vi "rs3 create frame queue.vi"(8 "error in (no error)":errorcluster, 11 "capacity":i32=2) -> (0 "error out":errorcluster, 1 "error":u64, 2 "queue":u64)   [LabVIEW 2017, in "libRealSense3.lvlib"]
doc: "Creates a Frame Queue that will be used to CAPTURE streams with. \nThis QUEUE goes into the START QUEUE and Wait_for_Frames VI.\n\nThe capacity should generally be at least as large as the number of streams configured to stream."
uses:
  libRealSense3.lvlib
  realsense2.dll
panel:
  # "RS3 Create Frame Queue"
  # "(C) Intel Corp.,  AGJ"
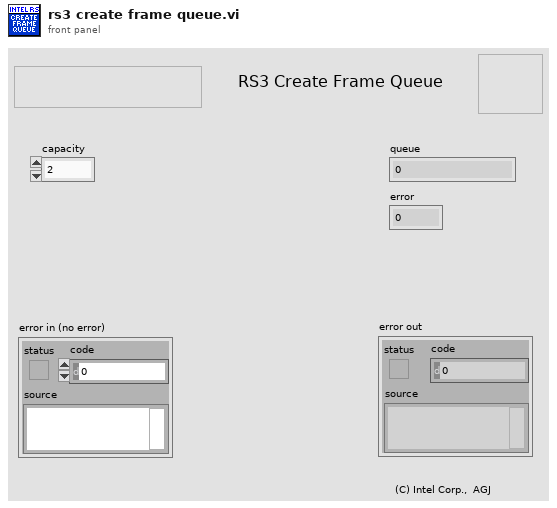
[diagram p1: front panel]
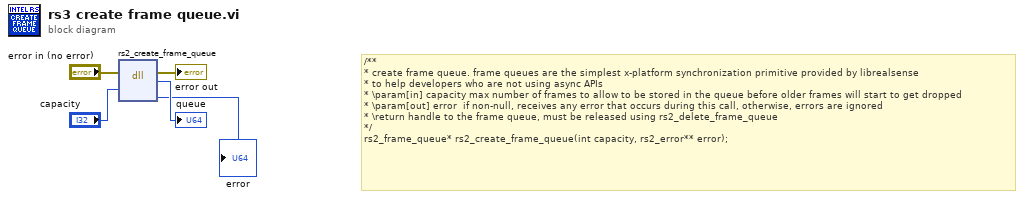
[diagram p0: block diagram]
diagram:
  # "/**\n* create frame queue. frame queues are the simplest x-platform synchronization primitive provided by librealsense\n* to help developers who are not using async APIs\n* \\param[in] capacity max number of frames to allow to be stored in the queue before older frames will start to get dropped\n* \\param[out] error  if non-null, receives any error that occurs during this call, otherwise, errors are ignored\n* \\return handle to the frame queue, must be released using rs2_delete_frame_queue\n*/\nrs2_frame_queue* rs2_create_frame_queue(int capacity, rs2_error** error);"
  n1 = dll-call lib="C:/Users/smartek/Desktop/labview/realsense2.dll" fn="rs2_create_frame_queue"(error in="error in (no error)", "capacity"="capacity") -> (error out=→"error out":errorcluster, "frame queue"=→"queue":u64, "error"=→"error":u64)  [unwired: 4 in, 1 out]
